vi "Read RIO Device Name.vi"(8 "error in (no error)":errorcluster, 11 "FPGA Device in":refnum<class "FPGA Device.lvclass">) -> (0 "error out":errorcluster, 2 "RIO Device Name":string, 3 "FPGA Device out":refnum<class "FPGA Device.lvclass">)   [LabVIEW 2016, in "FPGA RM Shared API.lvlib" / "FPGA Device.lvclass"]
uses:
  FPGA Device.lvclass
  FPGA Device.lvclass/FPGA Device.ctl
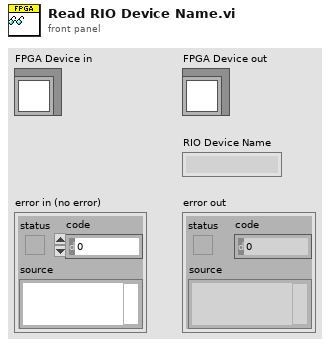
[diagram p1: front panel]
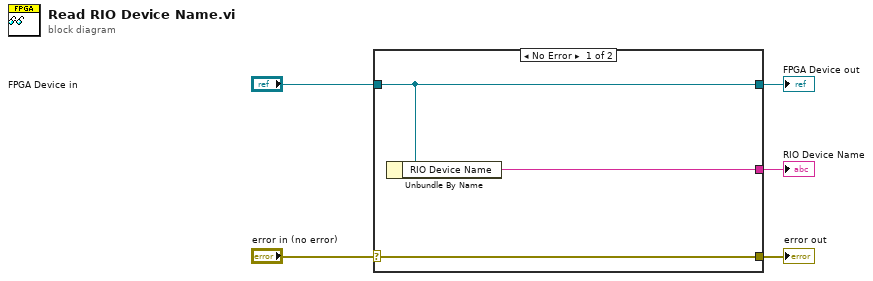
[diagram p0: block diagram]
diagram:
  n1 = case shown="No Error" "error in (no error)" {
    selector: "error in (no error)" -> [w8 w9]
    tunnel: [w8 w9] -> w4
    tunnel: [w7 w10] -> w2
    tunnel: "FPGA Device in" -> [w7 w10]
    tunnel: [w6 _] -> w1
    frame No Error {
      n2 = Unbundle By Name(w7) -> ("RIO Device Name"=w6:string)
    }
    frame Error {
    }
  }
  "error out" <- w4
  "FPGA Device out" <- w2
  "RIO Device Name" <- w1
